vi "Is Nested Typedef.vi"(8 "error in (no error)":errorcluster, 11 "object reference in":refnum<vi>) -> (0 "error out":errorcluster, 2 "is nested typedef?":bool, 3 "object reference out":refnum<vi>)   [LabVIEW 2020, in "MeasurementService Editor.lvlib"]
uses:
  MeasurementService Editor.lvlib
  a378e9ec-12ee-49ea-8886-5da9b61c1b52.vi
  2c171642-4819-4019-a916-92c127afeea5.vi
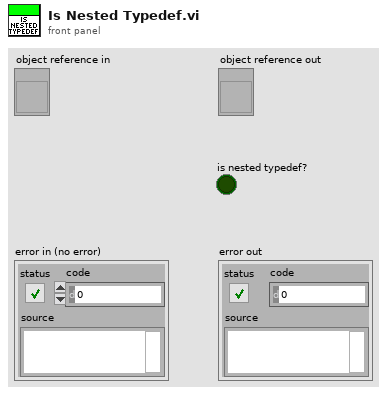
[diagram p1: front panel]
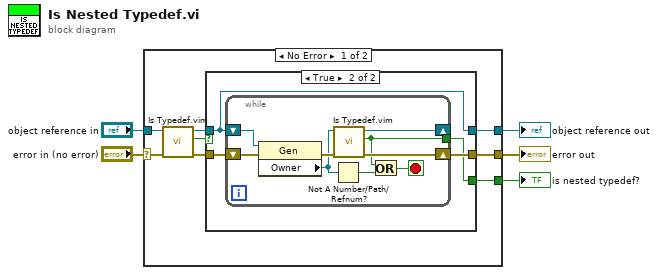
[diagram p0: block diagram]
diagram:
  n1 = case shown="No Error" "error in (no error)" {
    selector: "error in (no error)" -> [w12 w29]
    tunnel: "object reference in" -> [w13 w30]
    tunnel: [w8 w30] -> w4
    tunnel: [w7 w29] -> w3
    tunnel: [w6 _] -> w1
    frame No Error {
      n2 = call "Is Typedef.vim"("error in (no error)"=w12, "object reference in"=w13) -> ("error out"=w9:errorcluster, "is typedef?"=w11:bool, "object reference out"=w10:refnum<vi>)  [unwired: 7 in]
      n3 = case shown="True" w11 {
        tunnel: w10 -> [w15 w18]
        tunnel: w9 -> [w14 w19]
        tunnel: [w15 w18] -> w8
        tunnel: [w14 w17] -> w7
        tunnel: [_ w16] -> w6
        frame False {
        }
        frame True {
          n4 = while {
            shift-right: [w26] -> _
            shift-left: w18 -> [w28]
            shift-right: [w24] -> w17
            shift-left: w19 -> [w27]
            tunnel: [w20] -> w16
            stop <- w21 stop-if-true
            n5 = property class="Gen"(reference=w28, error in=w27) -> (error out=w25:errorcluster, "Owner"=w23:refnum<vi>)  [unwired: 1 out]
            n6 = Not A Number/Path/Refnum?(number/path/refnum=w23) -> (NaN/Path/Refnum?=w22:bool)
            n7 = call "Is Typedef.vim"("error in (no error)"=w25, "object reference in"=w23) -> ("error out"=w24:errorcluster, "is typedef?"=w20:bool, "object reference out"=w26:refnum<vi>)  [unwired: 7 in]
            n8 = Or(x=w20, y=w22) -> (x .or. y?=w21:bool)
          }
        }
      }
    }
    frame Error {
    }
  }
  "object reference out" <- w4
  "error out" <- w3
  "is nested typedef?" <- w1
